vi "LoadVarSetIntoVM.vi"(8 "error in (no error)":errorcluster, 10 "VarSet":T1, 11 "VariableManagerRef in":refnum<vi>) -> (0 "error out":errorcluster, 3 "VariableManagerRef out":refnum<vi>)   [LabVIEW 2013]
uses:
  FBVarSet.ctl
  FBVar.ctl
  VariableManagerCodes/VariableManager/VariableManager.lvclass
  VariableManagerCodes/Variable/Variable.lvclass
  VariableManagerCodes/API/VariableManagerAPI.lvlib
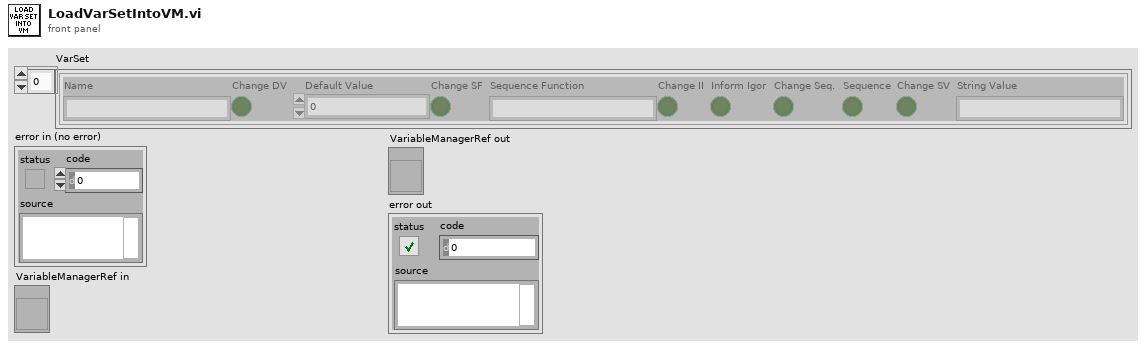
[diagram p1: front panel]
types:
  T1 = typedef "FBVarSet.ctl" = T2[]
  T2 = typedef "FBVar.ctl" = cluster{"Name":string, "Change DV":bool, "Default Value":dbl, "Change SF":bool, "Sequence Function":string, "Change II":bool, "Inform Igor":bool, "Change Seq.":bool, "Sequence":bool, "Change SV":bool, "String Value":string}
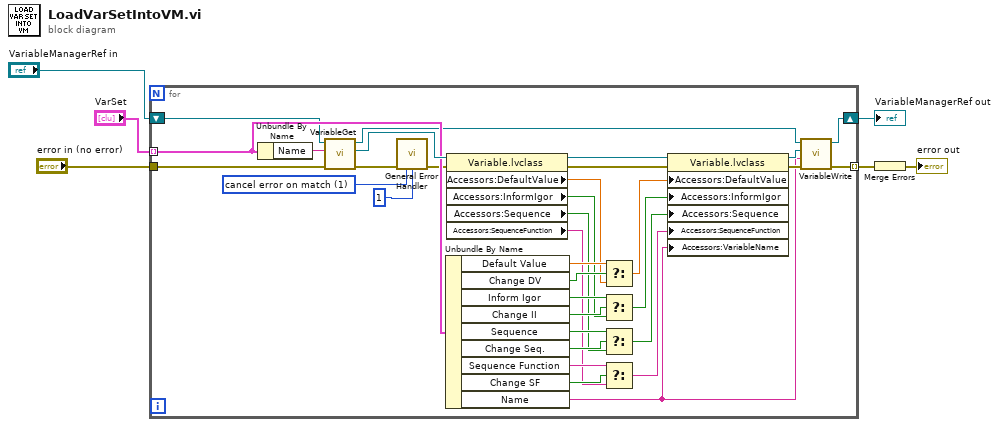
[diagram p0: block diagram]
diagram:
  n1 = for {
    tunnel: "VarSet" -> [w33] mode=indexing
    shift-right: [w9] -> w3
    shift-left: "VariableManagerRef in" -> [w8]
    tunnel: "error in (no error)" -> [w38]
    tunnel: [w10] -> w2 mode=indexing
    w37 = 1 items=["no exception", "cancel error on match", "set error on match"] ("[exception action] (none:0)")
    n2 = Unbundle By Name(w33) -> ("Name"=w39:string)
    n3 = call "VariableGet.vi"("error in (no error)"=w38, "VariableName"=w39, "VariableManagerRef in"=w8) -> ("error out"=w35:errorcluster, "Variable"=w34:refnum<class "Variable.lvclass">, "VariableManagerRef out"=w11:refnum<vi>)  [unwired: 6 in]
    n4 = call <vilib>:"General Error Handler.vi"("error in (no error)"=w35, "[exception action] (none:0)"=w37, "[exception code]"=1) -> ("error out"=w30:errorcluster)  [unwired: 8 in, 4 out]
    n5 = Unbundle By Name(w33) -> ("Default Value"=w27:dbl, "Change DV"=w26:bool, "Inform Igor"=w25:bool, "Change II"=w24:bool, "Sequence"=w23:bool, "Change Seq."=w22:bool, "Sequence Function"=w21:string, "Change SF"=w20:bool, "Name"=w7:string)
    n6 = property class="Variable.lvclass"(reference=w34, error in=w30) -> (reference out=w31:refnum<class "Variable.lvclass">, error out=w32:errorcluster, "Accessors:DefaultValue"=w19:dbl, "Accessors:InformIgor"=w18:bool, "Accessors:Sequence"=w17:bool, "Accessors:SequenceFunction"=w16:string)
    n7 = Select(t=w27, s=w26, f=w19) -> (s? t:f=w15:dbl)
    n8 = Select(t=w25, s=w24, f=w18) -> (s? t:f=w14:bool)
    n9 = Select(t=w23, s=w22, f=w17) -> (s? t:f=w13:bool)
    n10 = Select(t=w21, s=w20, f=w16) -> (s? t:f=w12:string)
    n11 = property class="Variable.lvclass"(reference=w31, error in=w32, "Accessors:DefaultValue"=w15, "Accessors:InformIgor"=w14, "Accessors:Sequence"=w13, "Accessors:SequenceFunction"=w12, "Accessors:VariableName"=w7) -> (reference out=w29:refnum<class "Variable.lvclass">, error out=w28:errorcluster)
    n12 = call "VariableWrite.vi"("error in (no error)"=w28, "OriginalName"=w7, "Variable"=w29, "VariableManagerRef in"=w11) -> ("error out"=w10:errorcluster, "VariableManagerRef out"=w9:refnum<vi>)  [unwired: 6 in]
  }
  "VariableManagerRef out" <- w3
  n13 = Merge Errors(w2) -> (→"error out":errorcluster)
